vi "Init_Test.vi"(8 "error in (no error)":errorcluster caption="entrée d'erreur (pas d'erreur)", 11 "Print_Label en entrée":refnum<class "Zigbee_Send_Command_UART.lvclass">) -> (0 "error out":errorcluster caption="sortie d'erreur", 3 "Print_Label en sortie":refnum<class "Zigbee_Send_Command_UART.lvclass">)   [LabVIEW 2020, in "Library Test.lvlib" / "Zigbee_Send_Command_UART.lvclass"]
uses:
  Zigbee_Send_Command_UART.lvclass
  C:/Users/ngarcin/OneDrive - Altyor/Standard TB/Class/Test/Test (Default)/Test (Default).lvclass
  Commun VI/TypeDef/Commande Test/Commande Value Type.ctl
  Commun VI/TypeDef/Commande Test/Commande Type Test.ctl
  Test_Wtih_Instr/Test_With_Inst.lvclass
  Instrument/Instrument (Default)/Class Instrument (Default).lvclass
  Zigbee_Send_Command_UART.lvclass/Zigbee_Send_Command_UART.ctl
  Commun VI/Library Commun.lvlib
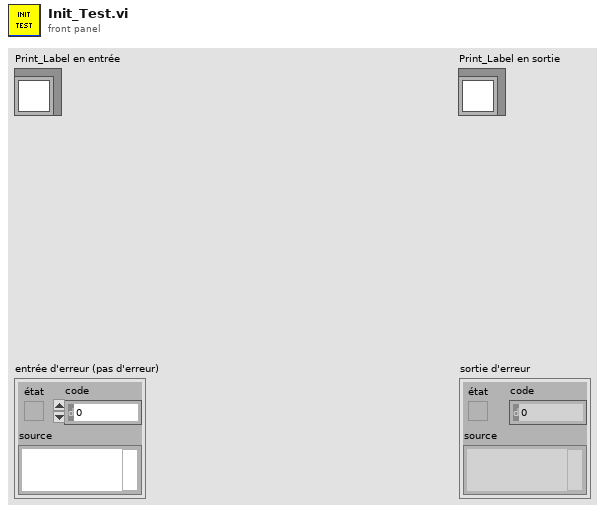
[diagram p1: front panel]
types:
  T1 = typedef "Library Commun.lvlib/Commande Type Test.ctl" = enum16{"Function", "Test", "Calculation"}
  T2 = typedef "Library Commun.lvlib/Commande Value Type.ctl" = enum16{"None", "String", "Number", "Timestamp", "Boolean", "Array"}
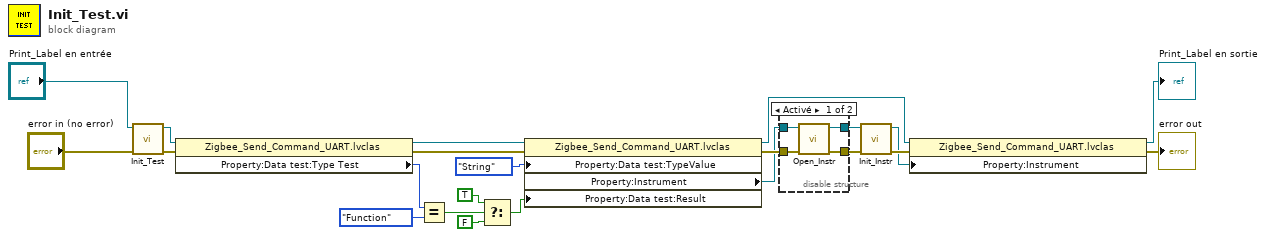
[diagram p0: block diagram]
diagram:
  n1 = call-parent "Init_Test.vi"("error in (no error)"="error in (no error)", "Test_With_Inst en entrée"="Print_Label en entrée") -> ("error out"=w10:errorcluster, "Test_With_Inst en sortie"=w8:refnum<class "Zigbee_Send_Command_UART.lvclass">)  [unwired: 8 in]
  n2 = property class="Zigbee_Send_Command_UART.lvclas"(reference=w8, error in=w10) -> (reference out=w7:refnum<class "Zigbee_Send_Command_UART.lvclass">, error out=w9:errorcluster, "Property:Data test:Type Test"=w6:T1)
  n3 = Equal?(x=w6, y=Commande_Type_Test."Function") -> (x = y?=w4:bool)
  n4 = Select(t=TRUE ("cas vrai"), s=w4, f=FALSE ("Result")) -> (s? t:f=w2:bool)
  n5 = property class="Zigbee_Send_Command_UART.lvclas"(reference=w7, error in=w9, "Property:Data test:TypeValue"=Commande_Value_Type."String" ("TypeValue"), "Property:Data test:Result"=w2) -> (reference out=w20:refnum<class "Zigbee_Send_Command_UART.lvclass">, error out=w16:errorcluster, "Property:Instrument"=w13:refnum<class "Class Instrument (Default).lvclass">)
  n6 = disable-structure shown="Activé" {
    disable-tunnel: w16 -> [w26 w27]
    disable-tunnel: [w25 w27] -> w15
    disable-tunnel: w13 -> [w24 w28]
    disable-tunnel: [w23 w28] -> w12
    frame Enabled {
      n7 = call-dynamic "Open_Instr.vi"("error in (no error)"=w26, "Class Multimeter (Default) en entrée"=w24) -> ("error out"=w25:errorcluster, "Class Multimeter (Default) en sortie"=w23:refnum<class "Class Instrument (Default).lvclass">)  [unwired: 8 in]
    }
    frame Disabled {
    }
  }
  n8 = call-dynamic "Init_Instr.vi"("error in (no error)"=w15, "Class Instrument (Default) en entrée"=w12) -> ("error out"=w14:errorcluster, "Class Instrument (Default) en sortie"=w11:refnum<class "Class Instrument (Default).lvclass">)  [unwired: 8 in]
  n9 = property class="Zigbee_Send_Command_UART.lvclas"(reference=w20, error in=w14, "Property:Instrument"=w11) -> (reference out=→"Print_Label en sortie":refnum<class "Zigbee_Send_Command_UART.lvclass">, error out=→"error out":errorcluster)
